vi "Set Output Lines.vi"(8 "Error In":errorcluster, 9 "Start Index":i32, 10 "DO Lines":bool[](array[boolean]), 11 "BNT_DAQmx-MCSV in":refnum<class "BNT_DAQmx-MCSV.lvclass">) -> (0 "Error Out":errorcluster, 3 "BNT_DAQmx-MCSV out":refnum<class "BNT_DAQmx-MCSV.lvclass">)   [LabVIEW 2020, in "BNT_DAQmx.lvlib" / "BNT_DAQmx-MCSV.lvclass"]
doc: "Write line values to DAQmx device and publish.\n\nTimeout is set to constant 1s."
uses:
  BNT_DAQmx-MCSV.lvclass
  BNT_DAQmx-MCSV.lvclass/BNT_DAQmx-MCSV.ctl
  <vilib>/DAQmx/write.llb/DAQmx Write (Digital 1D Bool NChan 1Samp 1Line).vi
  <vilib>/DAQmx/miscellaneous.llb/DAQmx Fill In Error Info.vi
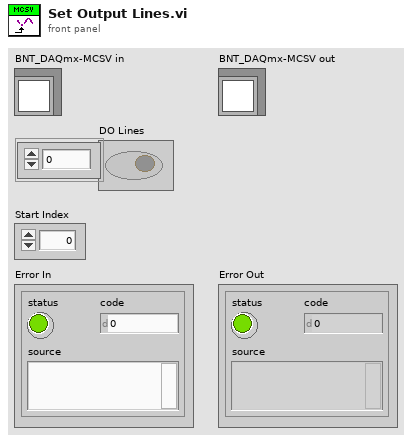
[diagram p1: front panel]
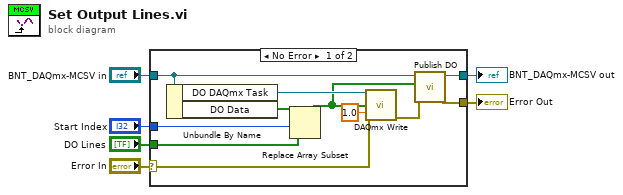
[diagram p0: block diagram]
diagram:
  n1 = case shown="No Error" "Error In" {
    selector: "Error In" -> [w15 w19]
    tunnel: [w7 w19] -> w5
    tunnel: [w11 w18] -> w3
    tunnel: "BNT_DAQmx-MCSV in" -> [w10 w18]
    tunnel: "DO Lines" -> [w13 _]
    tunnel: "Start Index" -> [w12 _]
    frame No Error {
      n2 = Unbundle By Name(w10) -> ("DO DAQmx Task"=w17:refnum<k21>, "DO Data"=w14:bool[])
      n3 = Replace Array Subset(array=w14, new element=w13, index=w12) -> (w9:bool[])
      n4 = call-poly <vilib>:"DAQmx Write.vi"("task/channels in"=w17, "data"=w9, "timeout"=1.0, "error in"=w15) -> ("error out"=w8:errorcluster)  [unwired: 9 in, 2 out]
      n5 = call "Publish DO.vi"("error in"=w8, "DO Data"=w9, "BNT_DAQmx-MCSV in"=w10) -> ("error out"=w7:errorcluster, "BNT_DAQmx-MCSV out"=w11:refnum<class "BNT_DAQmx-MCSV.lvclass">)  [unwired: 7 in]
    }
    frame Error {
    }
  }
  "Error Out" <- w5
  "BNT_DAQmx-MCSV out" <- w3
